vi "Dialog Scale name.vi"(0 "name in":string caption="Название датчика") -> (4 "name out":string, 6 "canceled":bool)   [LabVIEW 2019, in "GUI Sensor Lib.lvclass"]
uses:
  GUI Sensor Lib.lvclass
panel:
  in  "ok":bool
  in  "cancel":bool
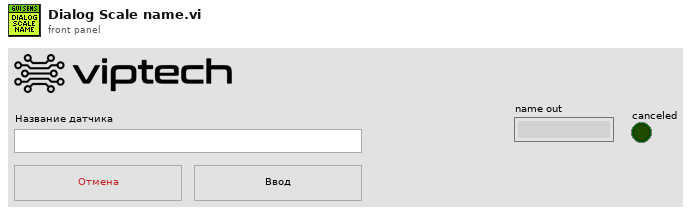
[diagram p1: front panel]
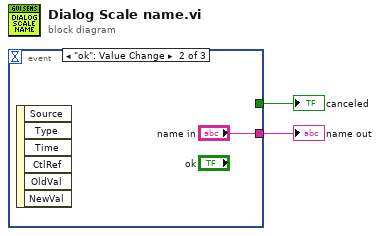
[diagram p0: block diagram]
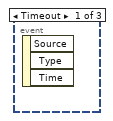
[diagram p2: hidden frame]
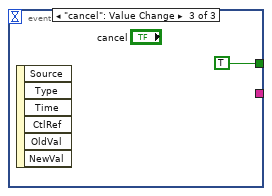
[diagram p3: hidden frame]
diagram:
  n1 = event shown="[1] \"ok\": Value Change" {
    selector: _ -> [_ _ _]
    dyn-events: _ -> [_ _ _]
    timeout: _ -> [_ _ _]
    tunnel: [_ "name in" _] -> w1
    tunnel: [_ _ TRUE] -> w2
    event Timeout {
      n2 = event-data() -> ()  [unwired: 1 in, 3 out]
    }
    event "ok": Value Change {
      n3 = event-data() -> ()  [unwired: 1 in, 6 out]
    }
    event "cancel": Value Change {
      n4 = event-data() -> ()  [unwired: 1 in, 6 out]
    }
  }
  "canceled" <- w2
  "name out" <- w1
